vi "CDAQ Index Array.vi"() -> (2 "CDAQ Index":string[][](array[string]))   [LabVIEW 2012]
panel:
  out "CDAQ Index Array":i32[](array[numeric])
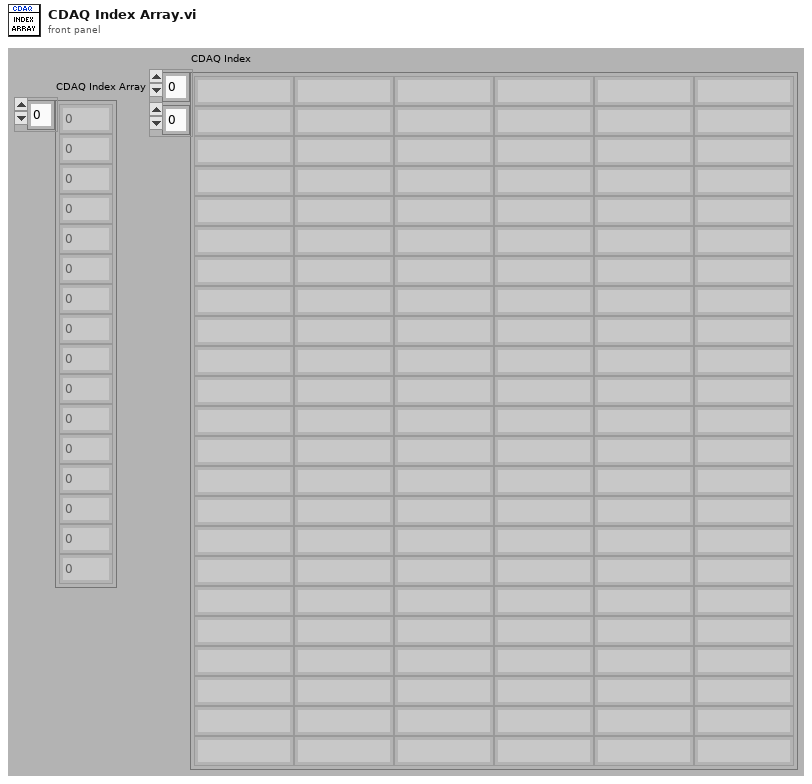
[diagram p1: front panel]
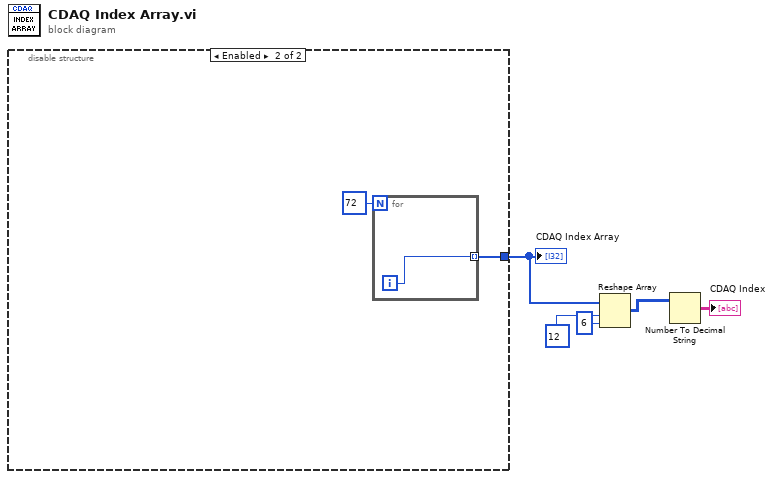
[diagram p0: block diagram]
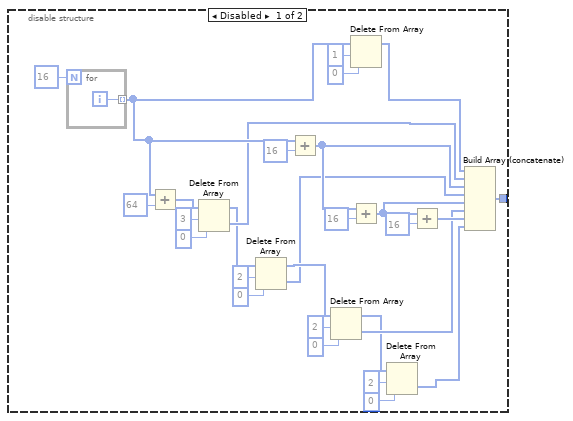
[diagram p2: hidden frame]
diagram:
  n1 = disable-structure shown="Enabled" {
    disable-tunnel: [w27 w36] -> w5
    frame Disabled {
      n2 = for {
        N: 16 -> [_]
        tunnel: [w35] -> w22 mode=indexing
        i -> [w35]
      }
      n3 = Add(x=w22, y=64 ("Numeric")) -> (x+y=w19:i32[])
      n4 = Delete From Array(array=w19, length=3, index=0) -> (deleted portion=w18:i32[], array with subset deleted=w15:i32[])
      n5 = Delete From Array(array=w15, length=2, index=0) -> (deleted portion=w6:i32[], array with subset deleted=w12:i32[])
      n6 = Add(x=w22, y=16 ("Numeric")) -> (x+y=w30:i32[])
      n7 = Delete From Array(array=w12, length=2, index=0) -> (deleted portion=w9:i32[], array with subset deleted=w8:i32[])
      n8 = Delete From Array(array=w22, length=1, index=0) -> (array with subset deleted=w26:i32[])  [unwired: 1 out]
      n9 = Add(x=w30, y=16 ("Numeric")) -> (x+y=w29:i32[])
      n10 = Delete From Array(array=w8, length=2, index=0) -> (deleted portion=w7:i32[])  [unwired: 1 out]
      n11 = Add(x=w29, y=16 ("Numeric")) -> (x+y=w28:i32[])
      n12 = Build Array (concatenate)(w26, w18, w30, w6, w29, w9, w28, w7) -> (w27:i32[])
    }
    frame Enabled {
      n13 = for {
        N: 72 -> [_]
        tunnel: [w38] -> w36 mode=indexing
        i -> [w38]
      }
    }
  }
  "CDAQ Index Array" <- w5
  n14 = Reshape Array(w5, 12 ("dimension size"), 6 ("dimension size")) -> (w2:i32[][])
  n15 = Number To Decimal String(number=w2) -> (decimal integer string=→"CDAQ Index":string[][])  [unwired: 1 in]
